vi "Init.vi"(8 "error in (no error)":errorcluster, 11 "UI Actor in":refnum<class "UI Actor.lvclass">) -> (0 "error out":errorcluster, 3 "UI Actor out":refnum<class "UI Actor.lvclass">)   [LabVIEW 2020, in "UI Actor.lvlib" / "UI Actor.lvclass"]
uses:
  UI Actor.lvclass
  C:/Program Files/National Instruments/LabVIEW 2020/vi.lib/ActorFramework/Actor/Actor.lvclass
  MSG/MSG.lvclass
  UI Actor.lvclass/UI Actor.ctl
  LHL Actor/LHL Actor.lvclass
  LHL Actor/LHL Actor.lvclass/LHL Actor.ctl
  MXN Actor/MXN Actor.lvclass
  MXN Actor/MXN Actor.lvclass/MXN Actor.ctl
  Quetzal Actor/Quetzal Actor.lvclass
  Quetzal Actor/Quetzal Actor.lvclass/Quetzal Actor.ctl
  MSG/MSG.lvclass/MSG.ctl
  Read Coins.vi
  Read Sub Panel Monedas.vi
  Read Productos .vi
  Read Sub Panel Prod.vi
  Read Sub Panel Mensajes.vi
  <vilib>/ActorFramework/Actor/Actor.lvclass
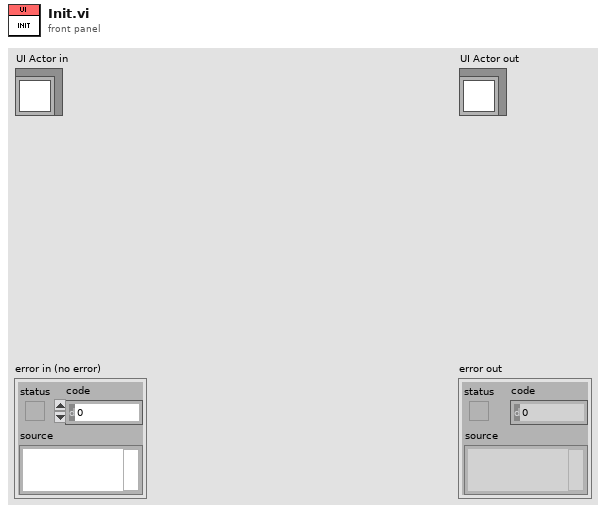
[diagram p1: front panel]
types:
  T1 = enum16{"La Hogaza de Lui", "MiniSuper Doña Rata"}
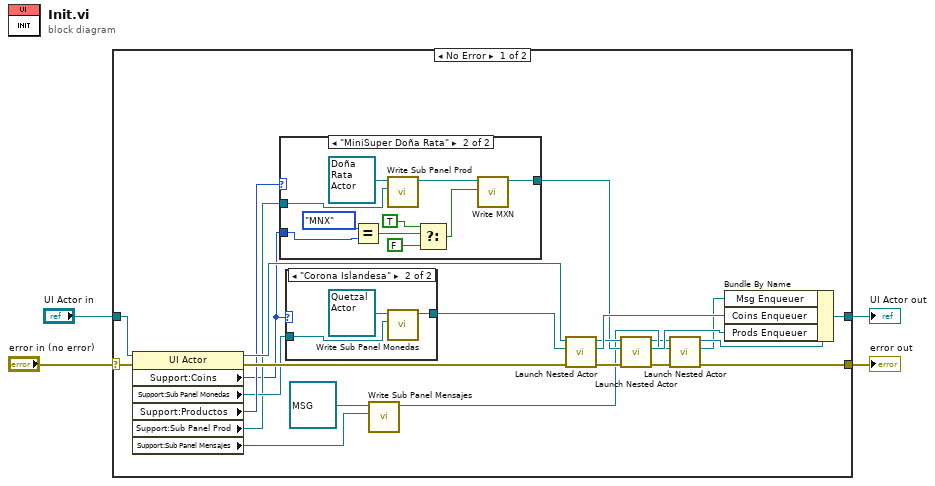
[diagram p0: block diagram]
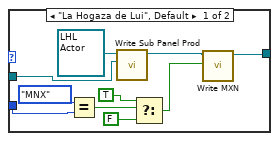
[diagram p2: hidden frame]
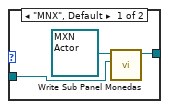
[diagram p3: hidden frame]
diagram:
  n1 = case shown="No Error" "error in (no error)" {
    selector: "error in (no error)" -> [w26 w55]
    tunnel: [w12 w55] -> w3
    tunnel: [w22 w54] -> w1
    tunnel: "UI Actor in" -> [w27 w54]
    frame No Error {
      n2 = property class="UI Actor"(reference=w27, error in=w26) -> (reference out=w23:refnum<class "UI Actor.lvclass">, error out=w25:errorcluster, "Support:Coins"=w5:enum16{"MNX", "Corona Islandesa"}, "Support:Sub Panel Monedas"=w19:refnum<vi>, "Support:Productos "=w20:T1, "Support:Sub Panel Prod"=w18:refnum<vi>, "Support:Sub Panel Mensajes"=w10:refnum<vi>)
      n3 = case shown="\"MiniSuper Doña Rata\"" w20 {
        tunnel: w18 -> [w36 w46]
        tunnel: [w29 w39] -> w15
        tunnel: w5 -> [w35 w41]
        frame "La Hogaza de Lui", Default {
          n4 = Equal?(x=enum16{"MNX", "Corona Islandesa"}."MNX", y=w35) -> (x = y?=w33:bool)
          n5 = call "Write Sub Panel Prod.vi"("Sub Panel Prod"=w36, "LHL Actor in"=refnum<class "LHL Actor.lvclass"> refnum ("LHL Actor.lvlib:LHL Actor.lvclass")) -> ("LHL Actor out"=w30:refnum<class "LHL Actor.lvclass">)  [unwired: 8 in, 1 out]
          n6 = Select(t=TRUE, s=w33, f=FALSE) -> (s? t:f=w28:bool)
          n7 = call "Write MXN.vi"("MXN"=w28, "LHL Actor in"=w30) -> ("LHL Actor out"=w29:refnum<class "LHL Actor.lvclass">)  [unwired: 8 in, 1 out]
        }
        frame "MiniSuper Doña Rata" {
          n8 = Equal?(x=enum16{"MNX", "Corona Islandesa"}."MNX", y=w41) -> (x = y?=w44:bool)
          n9 = call "Write Sub Panel Prod.vi"("Sub Panel Prod"=w46, "Doña Rata Actor in"=refnum<class "Doña Rata Actor.lvclass"> refnum ("Doña Rata Actor.lvlib:Doña Rata Actor.lvclass")) -> ("Doña Rata Actor out"=w40:refnum<class "Doña Rata Actor.lvclass">)  [unwired: 8 in, 1 out]
          n10 = Select(t=TRUE, s=w44, f=FALSE) -> (s? t:f=w38:bool)
          n11 = call "Write MXN.vi"("MXN"=w38, "Doña Rata Actor in"=w40) -> ("Doña Rata Actor out"=w39:refnum<class "Doña Rata Actor.lvclass">)  [unwired: 8 in, 1 out]
        }
      }
      n12 = case shown="\"Corona Islandesa\"" w5 {
        tunnel: [w49 w52] -> w24
        tunnel: w19 -> [w48 w51]
        frame "MNX", Default {
          n13 = call "Write Sub Panel Monedas.vi"("Sub Panel Monedas"=w48, "MXN Actor in"=refnum<class "MXN Actor.lvclass"> refnum ("MXN Actor.lvlib:MXN Actor.lvclass")) -> ("MXN Actor out"=w49:refnum<class "MXN Actor.lvclass">)  [unwired: 8 in, 1 out]
        }
        frame "Corona Islandesa" {
          n14 = call "Write Sub Panel Monedas.vi"("Sub Panel Monedas"=w51, "Quetzal Actor in"=refnum<class "Quetzal Actor.lvclass"> refnum ("Quetzal Actor.lvlib:Quetzal Actor.lvclass")) -> ("Quetzal Actor out"=w52:refnum<class "Quetzal Actor.lvclass">)  [unwired: 8 in, 1 out]
        }
      }
      n15 = call "Write Sub Panel Mensajes.vi"("Sub Panel Mensajes"=w10, "MSG in"=refnum<class "MSG.lvclass"> refnum ("MSG.lvlib:MSG.lvclass")) -> ("MSG out"=w9:refnum<class "MSG.lvclass">)  [unwired: 8 in, 1 out]
      n16 = call <vilib>:"Launch Nested Actor.vi"("error in (no error)"=w25, "Nested Actor"=w24, "Caller Actor in"=w23) -> ("error out"=w17:errorcluster, "Nested Actor's Enqueuer"=w21:refnum<class "Message Enqueuer.lvclass">, "Caller Actor out"=w16:refnum<class "UI Actor.lvclass">)  [unwired: 6 in]
      n17 = call <vilib>:"Launch Nested Actor.vi"("error in (no error)"=w17, "Nested Actor"=w15, "Caller Actor in"=w16) -> ("error out"=w13:errorcluster, "Nested Actor's Enqueuer"=w14:refnum<class "Message Enqueuer.lvclass">, "Caller Actor out"=w8:refnum<class "UI Actor.lvclass">)  [unwired: 6 in]
      n18 = call <vilib>:"Launch Nested Actor.vi"("error in (no error)"=w13, "Nested Actor"=w9, "Caller Actor in"=w8) -> ("error out"=w12:errorcluster, "Nested Actor's Enqueuer"=w6:refnum<class "Message Enqueuer.lvclass">, "Caller Actor out"=w7:refnum<class "UI Actor.lvclass">)  [unwired: 6 in]
      n19 = Bundle By Name(cluster=w7, "Msg Enqueuer"=w6, "Coins Enqueuer"=w21, "Prods Enqueuer"=w14) -> (w22:refnum<class "UI Actor.lvclass">)
    }
    frame Error {
    }
  }
  "error out" <- w3
  "UI Actor out" <- w1
